vi "Global_1259.vi"() -> ()   [LabVIEW 2018]
panel:
  out "BaseCurrent":string
  out "PowerMode":string
  in  "Inspection Point":string
  in  "Specsheet Scan":string
  in  "PO Line Number":string
  in  "PO Number":string
  in  "Inspector":string="id:0"
  in  "Station":string
  in  "EQF1259 com port":refnum<visa-resource-name>
  in  "Vendor Number":string
  in  "Vendor Name":string
  out "PIC_ARRAY":picture[](array[picture])=[bytes[1209480], bytes[921630], bytes[921630], bytes[346830], bytes[720330]]
  out "usbType":string
  out "Version":string[][](array[string])=[["Date", "Version", "Status", "Mod By"], ["20190701", "0", "Sic parvis magna", "id:0"], ["20191212", "1", "Successful test on 5 various consoles", "id:0"], ["20200125", "2", "Test for release", "id:0"], ["20200211", "3", "Fixed several bugs and rease for testing", "id:0"], ["20200213", "4", "Set foundation to handle Freemotion", "id:0"], ["20200214", "5", "Fixed small bugs", "id:0"], ["20200228", "6", "Changed reports so that all data will be visible with  SQL server", "id:0"], ["20200327", "-", "Release", "id:0"], ["20200331", "a", "Clean up of random indicators", "id:0"], ["20200407", "b", "Fixed instruction table", "id:0"], ["20200423", "c", "Added rower SPM and fixed verbiage", "id:0"], ["20200518", "d", "Modified some tests as per vendor suggestions", "id:0"], ["20200519", "e", "Noted treadmill issues fixed", "id:0"], ["20200520", "f", "Added resistance function for EBNT71017V1", "id:0"], ["20200522", "g", "Minor fixes and verbiage changes", "id:0"], ["20200810", "h", "Added wait for current to stablize in the audio tab...", "id:0"], ["20200909", "i", "Fixed feature and protocol scan for audio", "id:0"], ["20200919", "j", "Added wait for current to stablize after BLE test...", "id:0"], ["20201012", "k", "Removed audio automation and added steps for Kiwi consoles", "id:0"], ["20210121", "l", "Added Kiwi harness 1306 and 1309 steps...", ""]]
  in  "RS485_GearValues":dbl[][](array[numeric])=[[194.0, 245.0, 310.0, 375.0, 439.0, 504.0, 569.0, 634.0, 698.0, 763.0, 828.0, 892.0, 957.0, 1022.0, 1087.0, 1151.0, 1216.0, 1281.0, 1345.0, 1410.0, 1475.0, 1539.0, 0.0, 0.0], [194.0, 245.0, 310.0, 362.0, 427.0, 478.0, 543.0, 595.0, 659.0, 711.0, 776.0, 841.0, 892.0, 957.0, 1009.0, 1074.0, 1125.0, 1190.0, 1242.0, 1307.0, 1371.0, 1423.0, 1488.0, 1539.0], [207.0, 375.0, 556.0, 711.0, 892.0, 1048.0, 1203.0, 1384.0, 1552.0, 1734.0, 1889.0, 2070.0, 2225.0, 2381.0, 2458.0, 1229.0, 1384.0, 1565.0, 1734.0, 1915.0, 2070.0, 2251.0, 2407.0, 2458.0]]
  out "resistanceType":string
  out "gradeType":string
  out "speedType":string
  out "tabletType":string
  in  "KeyCodes":string[][](array[string])=[["1", "2", "3", "4", "5", "6", "7", "8", "9", "10", "11", "12", "13", "14", "15", "", "", "", "", "", "", "", "", "", "", "", "", "", "", "", "", "", "", "", "", "", "", "", "", "", "", "", "", "", "", "", "", "", "", "", "", "", "", "", "", "", "", "", "", "", ""], ["1", "2", "3", "4", "5", "6", "7", "8", "9", "10", "11", "12", "13", "14", "15", "16", "17", "18", "19", "20", "21", "22", "23", "24", "", "", "", "", "", "", "", "", "", "", "", "", "", "", "", "", "", "", "", "", "", "", "", "", "", "", "", "", "", "", "", "", "", "", "", "", ""], ["-20", "-19", "-18", "-17", "-16", "-15", "-14", "-13", "-12", "-11", "-10", "-9", "-8", "-7", "-6", "-5", "-4", "-3", "-2", "-1", "0", "1", "2", "3", "4", "5", "6", "7", "8", "9", "10", "11", "12", "13", "14", "15", "16", "17", "18", "19", "20", "21", "22", "23", "24", "25", "26", "27", "28", "29", "30", "31", "32", "33", "34", "35", "36", "37", "38", "39", "40"], ["0", "1", "2", "3", "4", "5", "6", "7", "8", "9", "10", "11", "12", "13", "14", "15", "16", "17", "18", "19", "20", "21", "22", "23", "24", "25", "26", "27", "28", "29", "30", "", "", "", "", "", "", "", "", "", "", "", "", "", "", "", "", "", "", "", "", "", "", "", "", "", "", "", "", "", ""], ["1", "2", "3", "4", "5", "6", "7", "8", "9", "10", "11", "12", "13", "14", "15", "16", "17", "18", "19", "20", "21", "22", "23", "24", "25", "26", "27", "28", "29", "30", "31", "32", "", "", "", "", "", "", "", "", "", "", "", "", "", "", "", "", "", "", "", "", "", "", "", "", "", "", "", "", ""]]
  out "maxCurrent":string
  out "runCurrent":string
  out "fanType":string
  out "CALIBRATE- 9":string
  out "distanceType":string
  out "FINISH-25":string
  out "WAHOO-22":string
  out "CSAFE-21":string
  out "TV-20":string
  out "AUDIO-19":string
  out "FAN-18":string
  out "PULSE-17":string
  out "USB-16":string
  out "RESISTANCE-15":string
  out "INCLINE-14":string
  out "RPM-13":string
  out "PWM-12":string
  out "MAINTENANCE MODE-8, 9, 10, 11":string
  out "BLE_CONNECT-7":string
  out "POWER_UP-5, 6":string
  out "COSMETIC-3, 4":string
  out "BLE_SETUP-2":string
  out "FIXTURE_SETUP-1":string
  out "NEEDED-0":string
  out "PIP_Instruction":string[][](array[string])
  out "unitType":string
  out "buttonType":string
  out "pulseType":string
  out "audioType":string
  out "ConsoleVoltage":string
  out "InclineMax":string
  out "InclineMin":string
  out "TransMax":string
  out "MaxSpeed":string
  out "tempNumeric":dbl
  out "tempBoolean":bool
  out "tempString":string
  out "displayType":string
  out "mcuType":string
  out "Firmware":string
  out "Controller/PowerBoard":string
  out "deviceType":string
  out "PartNumber":string
  out "Part Name":string
  out "TV":string
  out "DEMO":string
  out "WAHOO":string
  out "CSAFE":string
  out "TABLET":string
  out "PULSE":string
  out "RESISTANCE":string
  out "BLE":string
  out "BUZZER":string
  out "AUDIO":string
  out "FAN":string
  out "DISTANCE":string
  out "GRADE":string
  out "SPEED":string
  out "DMK":string
  out "USB":string
  # "byte[0]"
  # "Form Data"
  # "byte[1]"
  # "address: 0xA9 - 0xAA MPH; 0xAB - 0xAD KPH; 0xAE - 0xB6 INC; 0xB7 - 0xBA RES; 0xBB - 0xBE GEA"
  # "bytes |----------------------------------------|----------------------------------------|-----------------------------------------|----------------------------------------|----------------------------------------|----------------------------------------|-----------------------------------------|----------------------------------------|"
  # "*Use google translate and copy directly into here!"
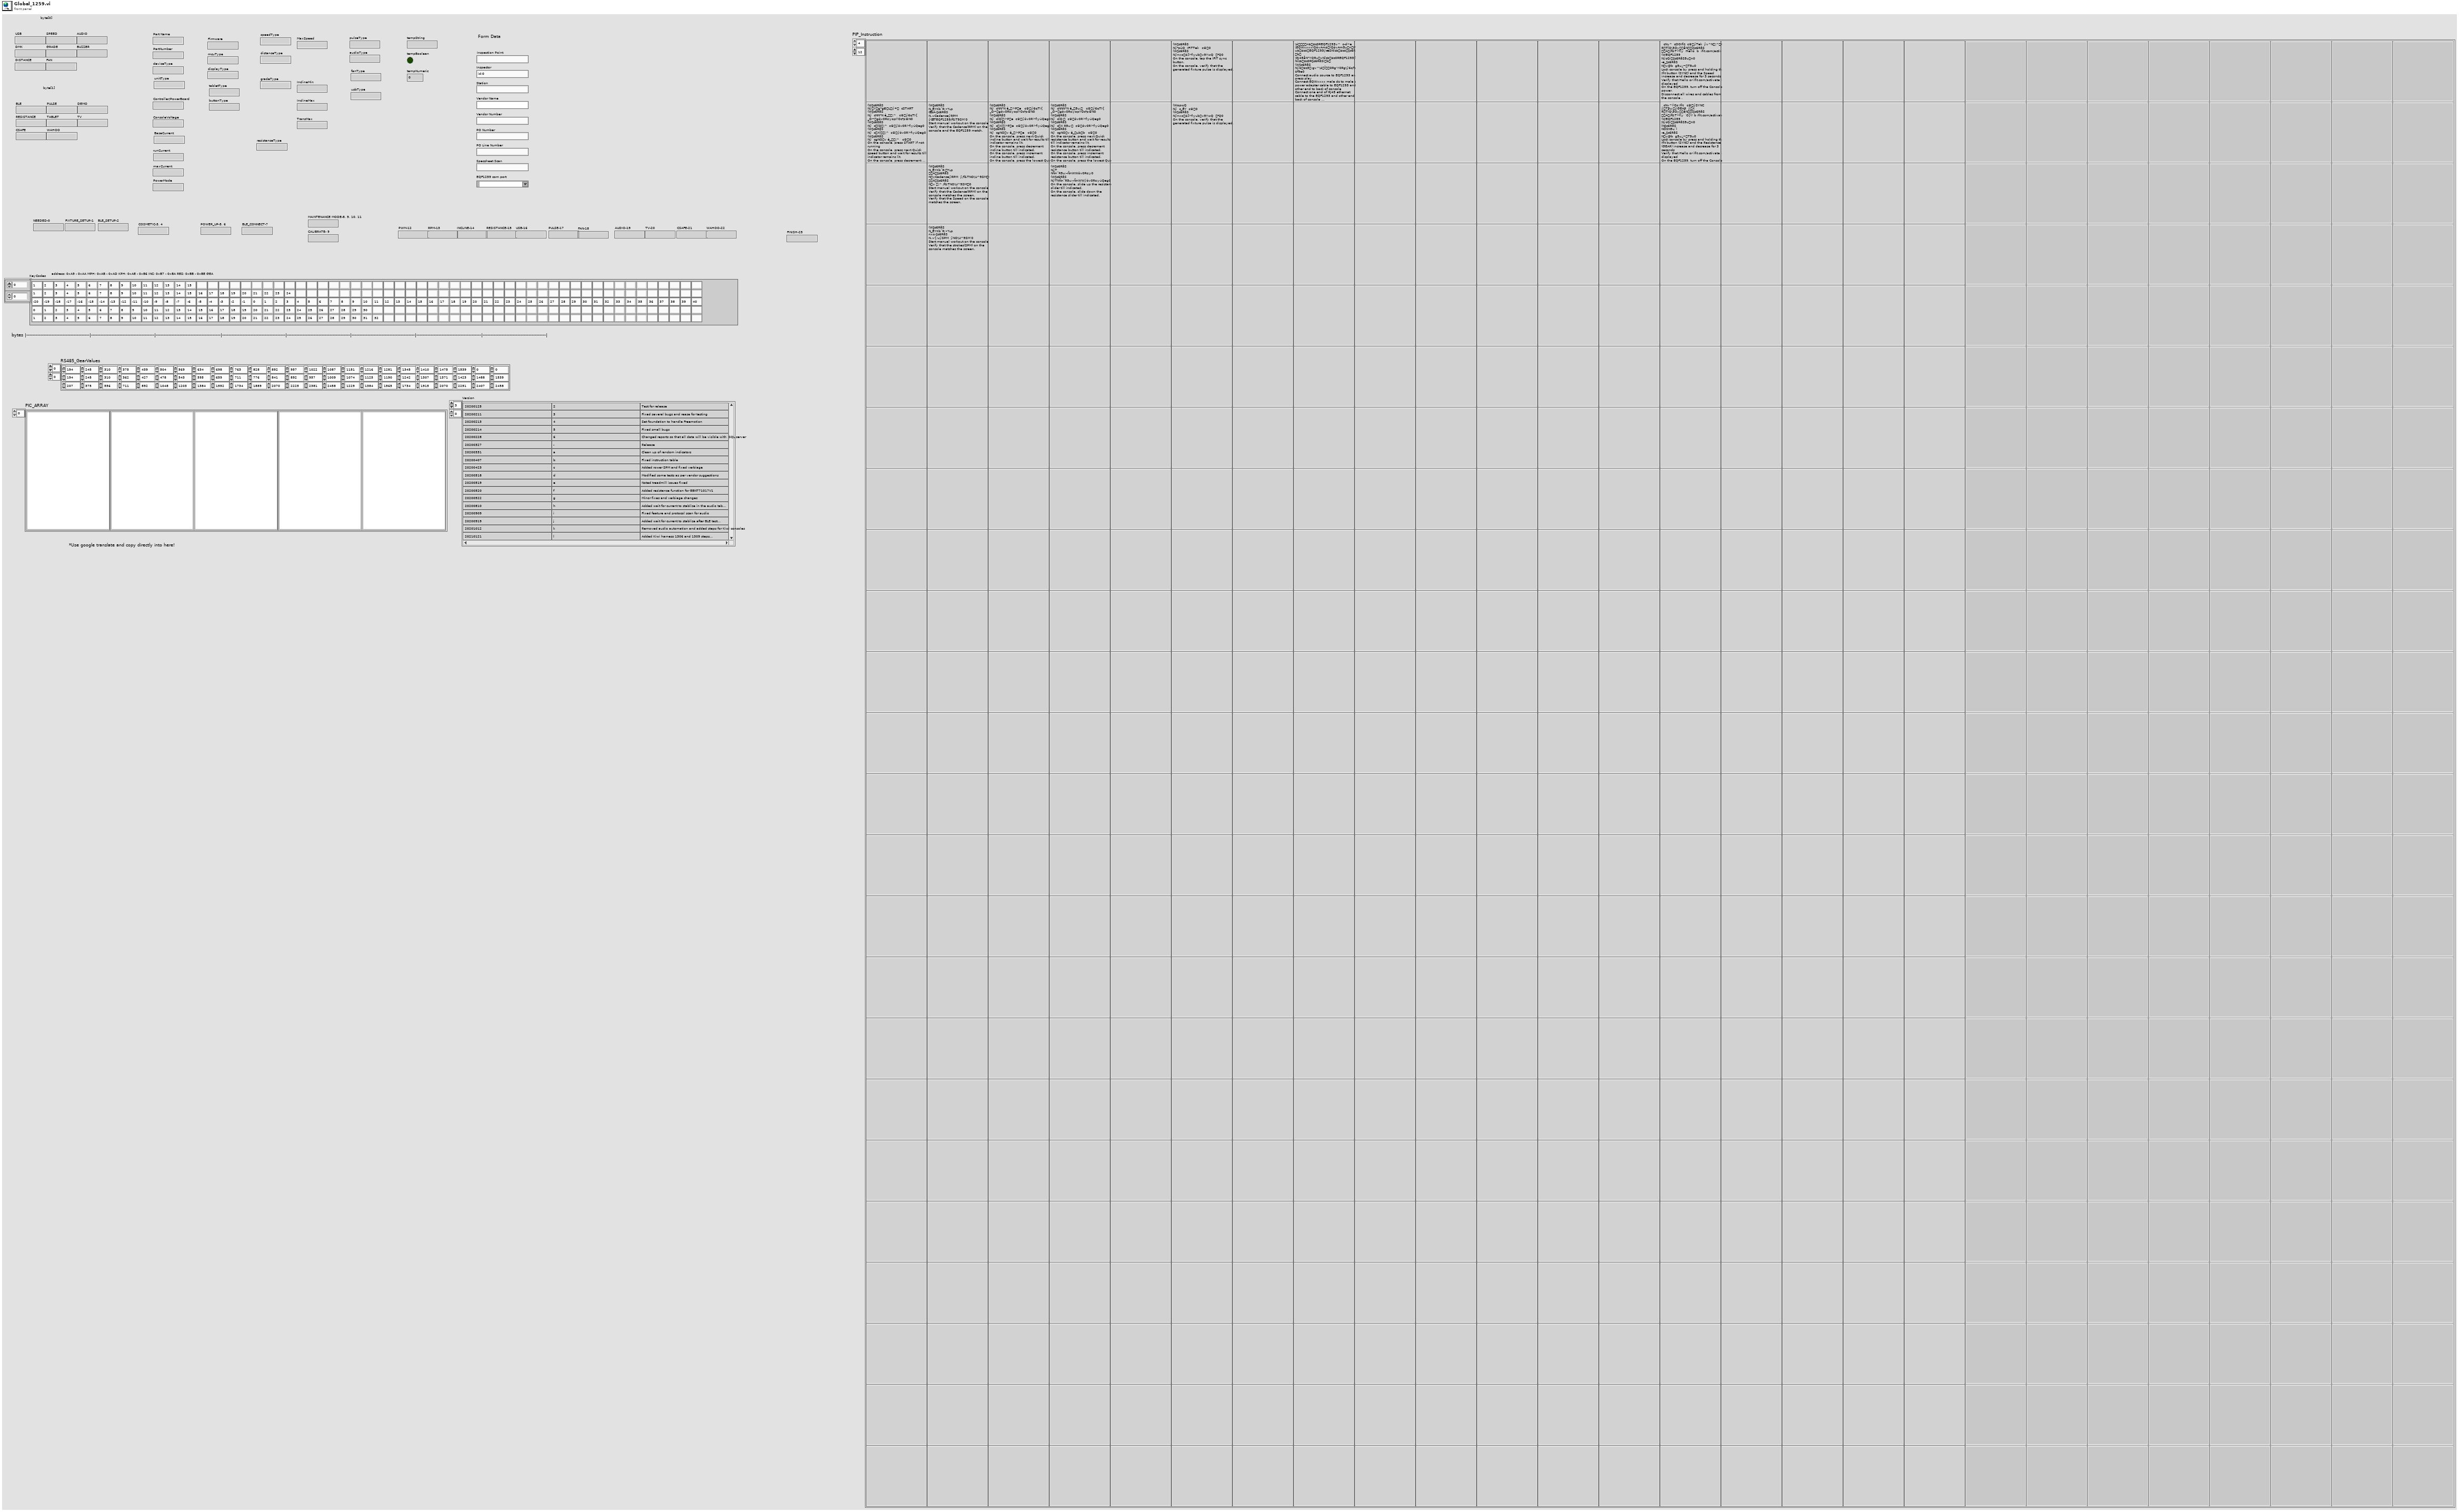
[diagram p1: front panel]
diagram:
